vi "Read.vi"   [LabVIEW 2015, in "Tektronix 7000 Series.lvlib"]
doc: "Initiates an acquisition on all channels that you enabled with the Configure Channel VI."
uses:
  Tektronix 7000 Series.lvlib
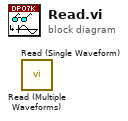
[diagram p0: block diagram]
diagram:
  n1 = call "Read (Multiple Waveforms).vi"() -> ()  [unwired: 9 in, 3 out]
  n2 = call "Read (Single Waveform).vi"() -> ()  [unwired: 9 in, 3 out]
